vi "test Get and Set Hardware Info.vi"(8 "error in (no error)":errorcluster, 11 "TestCase in":refnum<class "Framework Tests.lvclass">) -> (0 "error out":errorcluster, 3 "TestCase out":refnum<class "Framework Tests.lvclass">)   [LabVIEW 2017, in "Framework Tests.lvclass"]
uses:
  Framework Tests.lvclass
  Mock Framework Class/Mock Framework.lvclass
  C:/github/data-sharing-framework/Data Sharing Framework Core/Engine/Classes/Framework/Framework.lvclass
  Engine/Classes/Framework/Framework.lvclass/Framework.ctl
  <vilib>/addons/_JKI Toolkits/VI Tester/TestCase.llb/TestCase.lvclass
  Engine/Classes/Framework/Framework.lvclass
  Engine/Classes/Hardware/Hardware Info/Hardware Info.lvclass
  C:/Program Files (x86)/National Instruments/LabVIEW 2017/vi.lib/addons/_JKI Toolkits/VI Tester/TestCase.llb/TestCase.lvclass
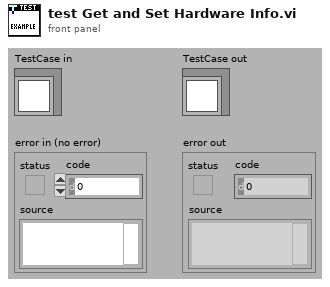
[diagram p1: front panel]
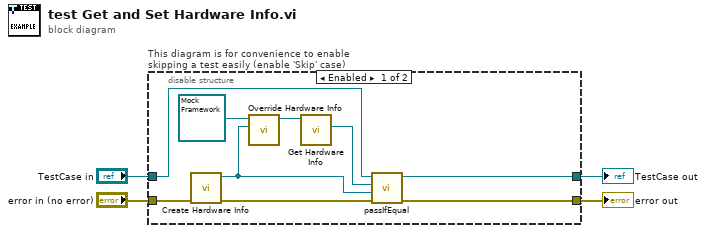
[diagram p0: block diagram]
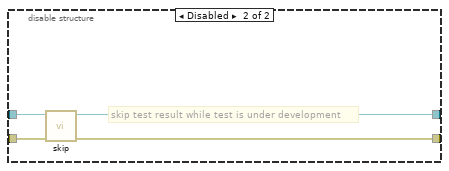
[diagram p2: hidden frame]
diagram:
  n1 = disable-structure "This diagram is for convenience to enable skipping a test easily (enable 'Skip' case)" shown="Enabled" {
    disable-tunnel: "TestCase in" -> [w12 w17]
    disable-tunnel: [w11 w15] -> w1
    disable-tunnel: [w13 w16] -> w2
    disable-tunnel: "error in (no error)" -> [w7 w14]
    frame Enabled {
      n2 = call "Create Hardware Info.vi"("error in (no error)"=w7) -> ("error out"=w6:errorcluster, "Hardware Info"=w5:refnum<class "Hardware Info.lvclass">)  [unwired: 9 in]
      n3 = call "Override Hardware Info.vi"("Hardware Info"=w5, "Mock Framework in"=refnum<class "Mock Framework.lvclass"> refnum) -> ("Mock Framework out"=w10:refnum<class "Mock Framework.lvclass">)  [unwired: 8 in, 1 out]
      n4 = call "Get Hardware Info.vi"("Framework in"=w10) -> ("Hardware Info"=w9:refnum<class "Hardware Info.lvclass">)  [unwired: 9 in, 1 out]
      n5 = call-dynamic "passIfEqual.vi"("error in (no error)"=w6, "y"=w5, "x"=w9, "TestCase in"=w12) -> ("error out"=w13:errorcluster, "TestCase out"=w11:refnum<class "Framework Tests.lvclass">)  [unwired: 6 in]
    }
    frame Disabled {
      # "skip test result while test is under development"
      n6 = call <vilib>:"skip.vi"("error in (no error)"=w14, "TestCase in"=w17) -> ("error out"=w16:errorcluster, "TestCase out"=w15:refnum<class "Framework Tests.lvclass">)  [unwired: 8 in]
    }
  }
  "error out" <- w2
  "TestCase out" <- w1
